vi "SDI Axis Straight Line.vi"() -> ()   [LabVIEW 2014]
uses:
  <vilib>/Motion/plugins/PluginFramework/nismSDIFramework.SetFrameworkMode.single.vi
  <vilib>/Motion/Express/_s/nimc.ex.clearFaults.clearFaults.axis.vi
  <vilib>/Motion/Express/_s/nimc.ex.power.power.axis.vi
  <vilib>/Motion/Express/_s/nimc.ex.read.readExecutionData.axis.vi
  <vilib>/Motion/Express/_s/nimc.ex.straightLineMove.startStraightLineMove.axis.modeAbsolute.0.vi
  <vilib>/Motion/Express/_s/nimc.ex.straightLineMove.startStraightLineMove.axis.modeRelative.0.vi
  <vilib>/Motion/Express/_s/nimc.ex.stopMove.stop.axis.modeDecelerate.vi
  <vilib>/Motion/BlockNode/FB.NIMotion.xnode
  <vilib>/Motion/plugins/SDI Plug-in - Delta ASDA/Template SoftMotion Drive Interface Plug-in Class.lvclass
panel:
  out "Example Done":bool
  out "error out":errorcluster
  in  "Stop Move":bool
  in  "Velocity":dbl=1000.0
  in  "Position":dbl=1000.0
  out "Move Position":cluster{"position":dbl, "velocity":dbl}(graph)={"position"=1000.0, "velocity"=0.0}
  in  "Move Mode":enum16{"Absolute", "Relative"}(ring)
  out "Move Done":bool
  in  "Resource":refnum<k21>="Axis 1"
  # "Move Constraints"
  # "Notes: \n1. This example uses preconfigured settings that may not be appropriate for your motion system. Review and update the axis settings using the Axis Configuration dialog box. Right-click each axis and select Properties to open the Axis Configuration dialog box. \n2. Running this example automatically activates all axes. Disable the \"Enable Drive on Transition to Active Mode\" option on the General Settings page of the Axis Configuration dialog box to prevent axes from activating when the VI runs.\n3. This example uses the default smoothing input to automatically calculate deceleration and jerk values. To specify these move constraints, connect a control to the \"smoothing\" input to adjust the value to your requirements. \n\nFor information about using this example in an actual motion system, refer to ni.com/info and enter Info Code nismex."
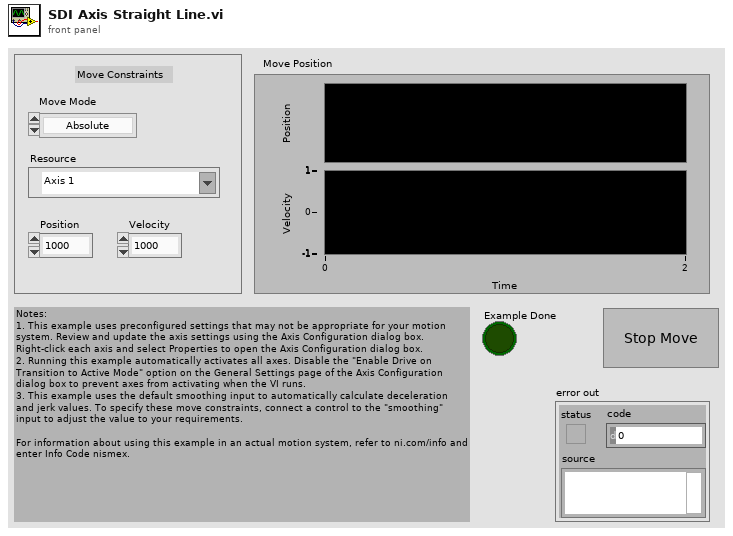
[diagram p1: front panel]
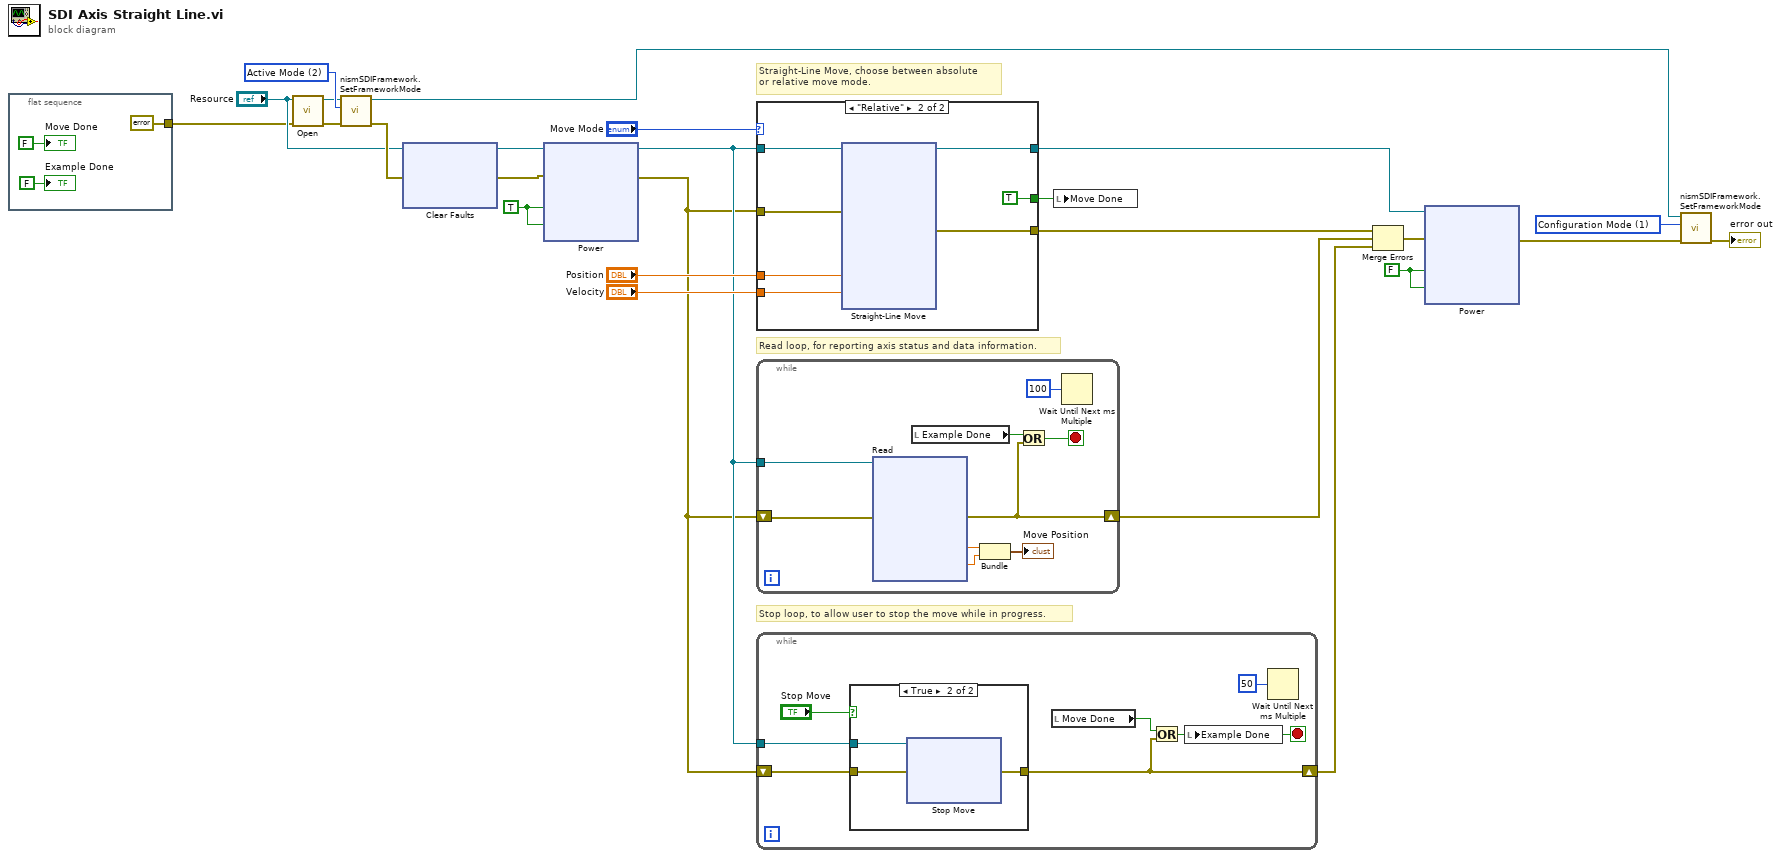
[diagram p0: block diagram]
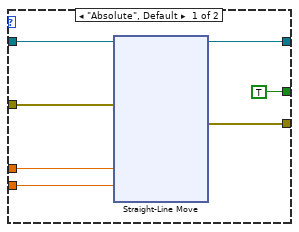
[diagram p3: hidden frame]
diagram:
  w10 = 1 items=["Configuration Mode"=1, "Active Mode"=2] ("mode (Active Mode)")
  w9 = FALSE ("enable axis")
  w15 = TRUE ("enable axis")
  w13 = 2 items=["Configuration Mode"=1, "Active Mode"=2] ("mode (Active Mode)")
  # "Read loop, for reporting axis status and data information."
  # "Stop loop, to allow user to stop the move while in progress."
  # "Straight-Line Move, choose between absolute\nor relative move mode."
  n1 = flat-sequence {
    tunnel: [errorcluster {"status"=FALSE, "code"=0, "source"=""} ("Error")] -> w3
    frame #0 {
      "Move Done" <- FALSE ("Example Done")
      "Example Done" <- FALSE
    }
  }
  n2 = call <vilib>:"Open.vi"("error in (no error)"=w3, "Axis"="Resource") -> ("error out"=w14:errorcluster, "Base Axis Out"=w12:refnum<class "nismPluginAxisBaseClass.lvclass">)  [unwired: 8 in]
  n3 = call-poly <vilib>:"nismSDIFramework.SetFrameworkMode.vi"("error in (no error)"=w14, "mode (Active Mode)"=w13, "Base Axis In"=w12) -> ("error out"=w16:errorcluster, "Base Axis Out"=w2:refnum<class "nismPluginAxisBaseClass.lvclass">)  [unwired: 7 in]
  n4 = xnode ("Clear Faults")("resource"="Resource", "error in"=w16) -> ("resource out"=w17:refnum<k21>, "error out"=w18:errorcluster)
  n5 = xnode ("Power")("enable axis"=w15, "enable drive"=w15, "resource"=w17, "error in"=w18) -> ("resource out"=w6:refnum<k21>, "error out"=w4:errorcluster)
  n6 = case shown="\"Relative\"" "Move Mode" {
    tunnel: w6 -> [w32 w54]
    tunnel: w4 -> [w35 w55]
    tunnel: [w31 w53] -> w19
    tunnel: "Position" -> [w34 w57]
    tunnel: "Velocity" -> [w33 w56]
    tunnel: [TRUE ("Example Done") TRUE] -> w20
    tunnel: [w29 w51] -> w1
    frame "Absolute", Default {
      n7 = xnode ("Straight-Line Move")("position"=w34, "velocity"=w33, "resource"=w32, "error in"=w35) -> ("resource out"=w29:refnum<k21>, "error out"=w31:errorcluster)  [unwired: 6 in, 1 out]
    }
    frame "Relative" {
      n8 = xnode ("Straight-Line Move")("position"=w57, "velocity"=w56, "resource"=w54, "error in"=w55) -> ("resource out"=w51:refnum<k21>, "error out"=w53:errorcluster)  [unwired: 6 in, 1 out]
    }
  }
  n9 = while {
    tunnel: w6 -> [w76]
    shift-right: [w75] -> w24
    shift-left: w4 -> [w73]
    stop <- w78 stop-if-true
    n10 = xnode ("Read")("resource"=w76, "error in"=w73) -> ("position"=w81:dbl, "velocity"=w80:dbl, "error out"=w75:errorcluster)  [unwired: 4 out]
    n11 = local read "Example Done"() -> (w77:bool)
    n12 = Bundle("position"=w81, "velocity"=w80) -> (→"Move Position":cluster{"position":dbl, "velocity":dbl})  [unwired: 1 out]
    n13 = Or(x=w77, y=w75) -> (x .or. y?=w78:bool)
    n14 = Wait Until Next ms Multiple(millisecond multiple=u32 100) -> ()  [unwired: 1 out]
  }
  n15 = while {
    tunnel: w6 -> [w95]
    shift-right: [w92] -> w21
    shift-left: w4 -> [w94]
    stop <- w91 stop-if-true
    n16 = case shown="True" "Stop Move" {
      tunnel: [w98 w101] -> w92
      tunnel: w95 -> [_ w100]
      tunnel: w94 -> [w98 w99]
      frame False {
      }
      frame True {
        n17 = xnode ("Stop Move")("resource"=w100, "error in"=w99) -> ("error out"=w101:errorcluster)  [unwired: 1 in, 2 out]
      }
    }
    n18 = local read "Move Done"() -> (w93:bool)
    n19 = Or(x=w93, y=w92) -> (x .or. y?=w91:bool)
    n20 = local write "Example Done"(w91) -> ()
    n21 = Wait Until Next ms Multiple(millisecond multiple=u32 50) -> ()  [unwired: 1 out]
  }
  n22 = local write "Move Done"(w20) -> ()
  n23 = Merge Errors(w19, w24, w21) -> (w8:errorcluster)
  n24 = xnode ("Power")("enable axis"=w9, "enable drive"=w9, "resource"=w1, "error in"=w8) -> ("error out"=w11:errorcluster)  [unwired: 1 out]
  n25 = call-poly <vilib>:"nismSDIFramework.SetFrameworkMode.vi"("error in (no error)"=w11, "mode (Active Mode)"=w10, "Base Axis In"=w2) -> ("error out"=→"error out":errorcluster)  [unwired: 7 in, 1 out]
